vi "save C scan image.vi"(9 "Image":picture, 10 "File name":string, 11 "Save Path":path=path "C:/Users/nbmlabgage/Desktop/LGD") -> ()   [LabVIEW 2014]
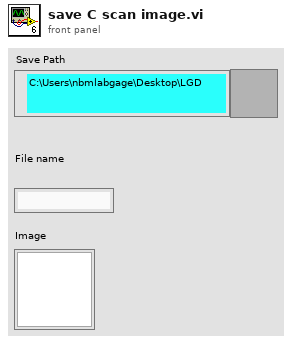
[diagram p1: front panel]
types:
  T1 = typedef "imagedata.ctl" = cluster{"image type":i32, "image depth":i32, "image":u8[], "mask":u8[], "colors":u32[], "Rectangle":cluster{"left":i16, "top":i16, "right":i16, "bottom":i16}}
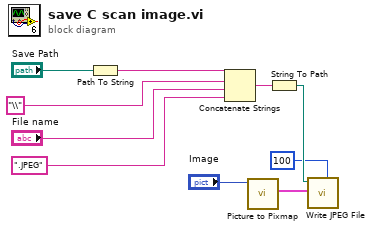
[diagram p0: block diagram]
diagram:
  n1 = Path To String(path="Save Path") -> (string=w9:string)
  n2 = Concatenate Strings(w9, "\\" ("string"), "File name", ".JPEG" ("string")) -> (w4:string)
  n3 = call <vilib>:"Picture to Pixmap.vi"("picture"="Image") -> ("image data"=w5:T1)  [unwired: 9 in, 1 out]
  n4 = String To Path(string=w4) -> (path=w3:path)
  n5 = call <vilib>:"Write JPEG File.vi"("quality (80)"=100, "image data"=w5, "path to JPEG file"=w3) -> ()  [unwired: 7 in, 2 out]
